vi "Read DC Pins.vi"(8 "error in (no error)":errorcluster, 11 "DCPower in":refnum<class "DCPower.lvclass">) -> (0 "error out":errorcluster, 2 "DC Pins":string[](array[string]), 3 "DCPower out":refnum<class "DCPower.lvclass">)   [LabVIEW 2018, in "DCPower.lvlib" / "DCPower.lvclass"]
uses:
  DCPower.lvclass
  DCPower.lvclass/DCPower.ctl
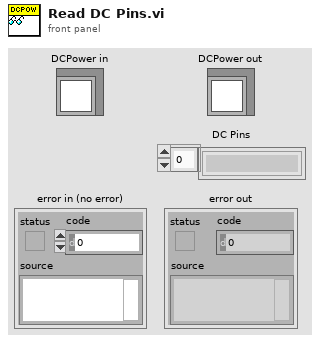
[diagram p1: front panel]
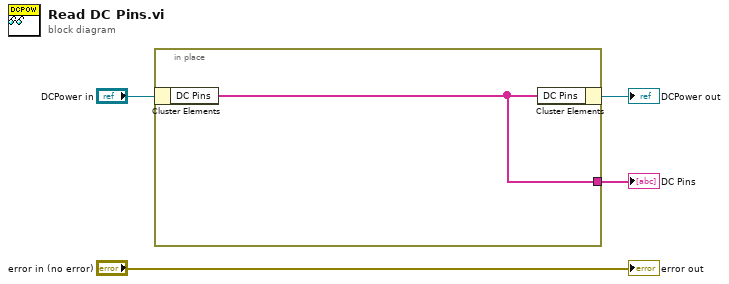
[diagram p0: block diagram]
diagram:
  n1 = in-place {
    in-place-border: [w5] -> w1
    n2 = in-place-cluster #1("DCPower in") -> ("DC Pins"=w5:string[])
    n3 = in-place-cluster #1("DC Pins"=w5) -> (→"DCPower out":refnum<class "DCPower.lvclass">)
  }
  "DC Pins" <- w1
  "error out" <- "error in (no error)"
